vi "dfd_Check Input (1D).vi"(8 "error in (no error)":errorcluster, 11 "x":dbl[](array[numeric])) -> (0 "error out":errorcluster, 3 "dup x":dbl[](array[numeric]))   [LabVIEW 2017, in "NI_DigFilter_Process.lvlib"]
uses:
  <vilib>/addons/Digital Filter Design/NI_DigFilter_Process.lvlib
  <vilib>/addons/Digital Filter Design/_Misc.llb/dfd_Error Handlers (Single).vi
  <vilib>/addons/Digital Filter Design/NI_DigFilterLicensed.lvlib
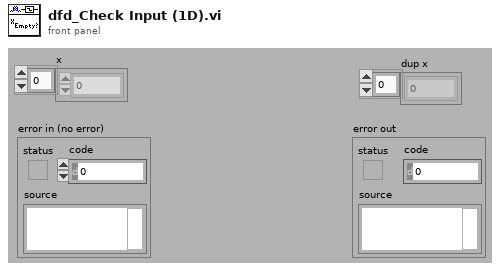
[diagram p1: front panel]
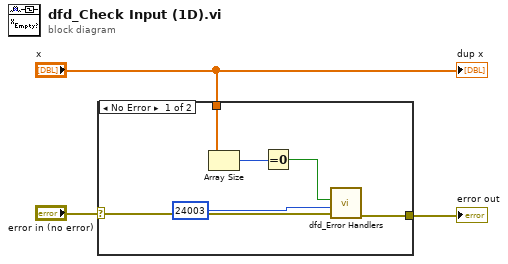
[diagram p0: block diagram]
diagram:
  n1 = case shown="No Error" "error in (no error)" {
    selector: "error in (no error)" -> [w6 w10]
    tunnel: [w9 w10] -> w3
    tunnel: "x" -> [w5 _]
    frame No Error {
      n2 = Array Size(array=w5) -> (size(s)=w7:i32)
      n3 = Equal To 0?(x=w7) -> (x = 0?=w4:bool)
      n4 = call-poly <vilib>:"dfd_Error Handlers.vi"("error in (no error)"=w6, "error code"=24003 ("WRN_#INPUT_ZERO"), "condition failed?"=w4) -> ("error out"=w9:errorcluster)  [unwired: 8 out]
    }
    frame Error {
    }
  }
  "error out" <- w3
  "dup x" <- "x"
